vi "MTM2_cancelCallback_command_clearErrors.vi"(8 "error in (no error)":errorcluster) -> (0 "error out":errorcluster, 3 "function return":i32)   [LabVIEW 2018, in "SALLV_MTM2.lvlib"]
doc: "int MTM2_shm_cancelCallback_command_clearErrorsLV();"
uses:
  SALLV_MTM2.lvlib
  SALLV_MTM2.so
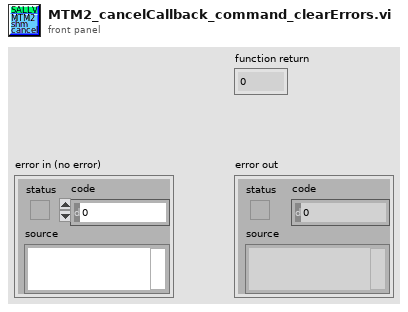
[diagram p1: front panel]
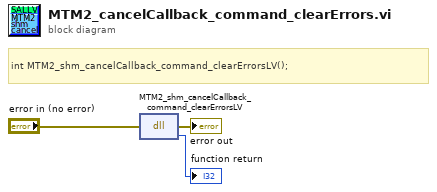
[diagram p0: block diagram]
diagram:
  # "int MTM2_shm_cancelCallback_command_clearErrorsLV();"
  n1 = dll-call lib="home/ttsai/Documents/salTestLabViewApi/SALLV_MTM2/SALLV_MTM2.*" fn="MTM2_shm_cancelCallback_command_clearErrorsLV"(error in="error in (no error)") -> (error out=→"error out":errorcluster, →"function return":i32)  [unwired: 2 in, 1 out]
